vi "WritePowerEnergy.vi"(1 "本次文件名":string) -> ()   [LabVIEW 2018]
uses:
  Init/AllPath.vi
  Reslut.vi
  <vilib>/Utility/file.llb/Write Delimited Spreadsheet (string).vi
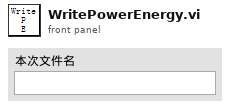
[diagram p1: front panel]
types:
  T1 = cluster{"能量计结果":string, "功率计结果":string, "能量计单位":string, " 功率计单位":string}
  T2 = cluster{"激光器型号":string, "X":dbl, "Y":dbl, "Z":dbl, "Rotate":dbl, "Pitching":dbl}
  T3 = cluster{"能量/功率":path, " 示波器":path, " 光谱仪":path, "偏振":path, "近远场":cluster{" 近场图片":path, " 远场图片":path, "发散角数据":path}, "参数":path, " 基路径":path, "文件名信息":path}
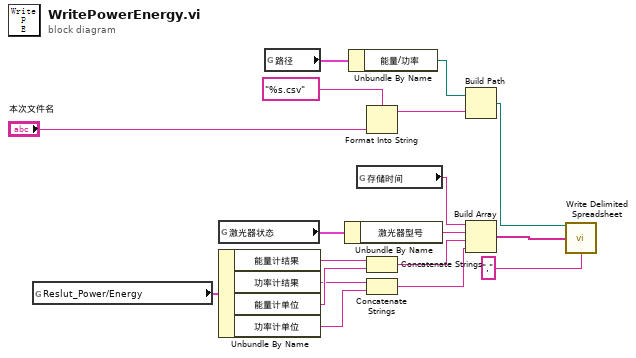
[diagram p0: block diagram]
diagram:
  n1 = global read "Reslut.vi" "Reslut_Power/Energy"() -> (w15:T1)
  n2 = global read "参数.vi" "激光器状态"() -> (w16:T2)
  n3 = Unbundle By Name(w15) -> ("能量计结果"=w14:string, "功率计结果"=w12:string, "能量计单位"=w13:string, "功率计单位"=w11:string)
  n4 = global read "AllPath.vi" "路径"() -> (w18:T3)
  n5 = Unbundle By Name(w16) -> ("激光器型号"=w1:string)
  n6 = Unbundle By Name(w18) -> ("能量/功率"=w17:path)
  n7 = global read "Reslut.vi" "存储时间"() -> (w2:string)
  n8 = Format Into String(format string="%s.csv" ("格式字符串"), "本次文件名") -> (resulting string=w3:string)  [unwired: 2 in, 1 out]
  n9 = Concatenate Strings(w14, w13) -> (w10:string)
  n10 = Concatenate Strings(w12, w11) -> (w9:string)
  n11 = Build Path(base path=w17, name or relative path=w3) -> (appended path=w7:path)
  n12 = Build Array(w2, w1, w10, w9) -> (w8:string[])
  n13 = call-poly <vilib>:"Write Delimited Spreadsheet.vi"("file path (dialog if empty)"=w7, "1D data"=w8, "delimiter (\\t)"="," ("delimiter (\\t)")) -> ()  [unwired: 11 in, 2 out]
